vi "Axis modifications.vi"(1 "Driver JoyStick Info":cluster{"Slow Drive?":bool, "Axisses":dbl[]}) -> (0 "Driver JoyStick Info Out":cluster{"Slow Drive?":bool, "Axisses":dbl[]})   [LabVIEW 2012]
uses:
  Drive Global Data.vi
panel:
  # "Out"
  # "In"
  # "X"
  # "Y"
  # "X"
  # "Y"
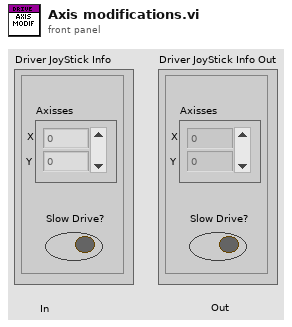
[diagram p1: front panel]
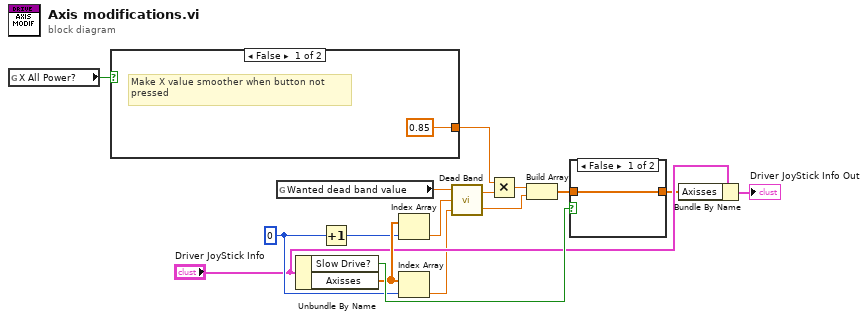
[diagram p0: block diagram]
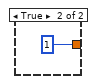
[diagram p2: hidden frame]
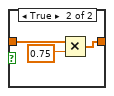
[diagram p3: hidden frame]
diagram:
  w13 = 0 ("index")
  n1 = global read "Drive Global Data.vi" "X All Power?"() -> (w1:bool)
  n2 = case shown="False" w1 {
    tunnel: [0.85 1] -> w2
    frame False {
      # "Make X value smoother when button not \npressed"
    }
    frame True {
    }
  }
  n3 = global read "Drive Global Data.vi" "Wanted dead band value"() -> (w5:dbl)
  n4 = Unbundle By Name("Driver JoyStick Info") -> ("Slow Drive?"=w16:bool, "Axisses"=w15:dbl[])
  n5 = Increment(x=w13) -> (x+1=w14:i32)
  n6 = Index Array(array=w15, index=w14) -> (element=w4:dbl)
  n7 = Index Array(array=w15, index=w13) -> (element=w3:dbl)
  n8 = call "Dead Band.vi"("Axis 2 In"=w3, "Axis 1 In"=w4, "Dead Band"=w5) -> ("Axis 2 Out"=w6:dbl, "Axis 1 Out"=w7:dbl)
  n9 = Multiply(x=w2, y=w7) -> (x*y=w10:dbl)
  n10 = Build Array(w10, w6) -> (w9:dbl[])
  n11 = case shown="False" w16 {
    tunnel: [w19 w21] -> w8
    tunnel: w9 -> [w19 w20]
    frame False {
    }
    frame True {
      n12 = Multiply(x=w20, y=0.75) -> (x*y=w21:dbl[])
    }
  }
  n13 = Bundle By Name(cluster="Driver JoyStick Info", "Axisses"=w8) -> (→"Driver JoyStick Info Out":cluster{"Slow Drive?":bool, "Axisses":dbl[]})
